vi "_get control reference by name.vi"(4 "error in (no error)":errorcluster, 5 "Control name":string, 6 "Case sensitive (T)":bool, 7 "Control references":cluster{string, refnum<vi>}[](array[cluster])) -> (0 "error out":errorcluster, 2 "Ctl Refnum":refnum<vi>)   [LabVIEW 2019]
doc: "This VI will give you a control refrence by feeding it the output of the\" get reference to all controls\" VI and the name of the control you would like a reference to."
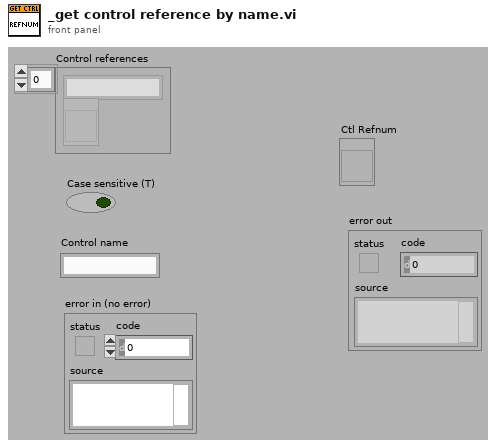
[diagram p1: front panel]
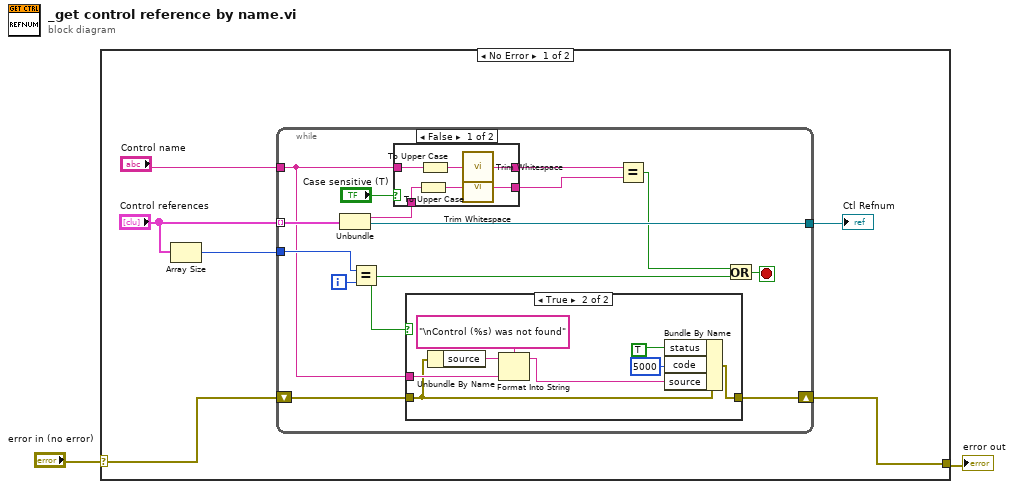
[diagram p0: block diagram]
diagram:
  n1 = case shown="No Error" "error in (no error)" {
    selector: "error in (no error)" -> [w5 w40]
    tunnel: [w4 w40] -> w2
    frame No Error {
      n2 = Array Size(array="Control references") -> (size(s)=w8:i32)
      n3 = while {
        tunnel: "Control references" -> [w22] mode=indexing
        tunnel: [w21] -> w6
        tunnel: "Control name" -> [w9]
        tunnel: w8 -> [w19]
        shift-right: [w10] -> w4
        shift-left: w5 -> [w11]
        i -> [w20]
        stop <- w17 stop-if-true
        n4 = Unbundle(w22) -> (w14:string, w21:refnum<vi>)
        n5 = Equal?(x=w19, y=w20) -> (x = y?=w16:bool)
        n6 = case shown="False" "Case sensitive (T)" {
          tunnel: w9 -> [w23 w30]
          tunnel: w14 -> [w28 w29]
          tunnel: [w27 w30] -> w13
          tunnel: [w25 w29] -> w12
          frame False {
            n7 = To Upper Case(1:w28) -> (0:w26:string)
            n8 = To Upper Case(1:w23) -> (0:w24:string)
            n9 = call <vilib>:"Trim Whitespace.vi"("string"=w24) -> ("trimmed string"=w27:string)  [unwired: 1 in]
            n10 = call <vilib>:"Trim Whitespace.vi"("string"=w26) -> ("trimmed string"=w25:string)  [unwired: 1 in]
          }
          frame True {
          }
        }
        n11 = case shown="True" w16 {
          tunnel: w11 -> [w31 w33]
          tunnel: [w31 w39] -> w10
          tunnel: w9 -> [_ w38]
          frame False {
          }
          frame True {
            n12 = Unbundle By Name(w33) -> ("source"=w32:string)
            n13 = Format Into String(format string="\nControl (%s) was not found", initial string=w32, w38) -> (resulting string=w36:string)  [unwired: 1 in, 1 out]
            n14 = Bundle By Name(cluster=w33, "status"=TRUE ("Error/Warning"), "code"=5000, "source"=w36) -> (w39:errorcluster)
          }
        }
        n15 = Equal?(x=w13, y=w12) -> (x = y?=w18:bool)
        n16 = Or(x=w18, y=w16) -> (x .or. y?=w17:bool)
      }
      "Ctl Refnum" <- w6
    }
    frame Error {
    }
  }
  "error out" <- w2
